vi "Teleop.vi"(10 "Match Info":T1={"Autonomous Elapsed Seconds"=0.0, "TeleOp Elapsed Seconds"=0.0, "Disabled Elapsed Seconds"=0.0, "Visited Autonomous"=FALSE, "Visited TeleOp"=FALSE, "Visited Disabled"=FALSE, "Autonomous Settings"={"Autonomous Style"=enum."Independent", "VI Refnum"=refnum}}, 11 "Call Context":T2) -> ()   [LabVIEW 2014]
doc: "This VI is called for each TeleOp packet received from the DS where the robot is not disabled. It is often used to read from the joysticks and update I/O or to update setpoints for timed control loops. It should complete and return within 20 milliseconds or it may miss DS packets."
uses:
  <vilib>/Rock Robotics/WPI/DriverStation/WPI_DriverStationDerivedRobotMode.ctl
  <vilib>/Rock Robotics/WPI/DriverStation/WPI_DriverStationMatch Info.ctl
  <vilib>/Rock Robotics/WPI/Joystick/WPI_JoystickGetSetRefNum.vi
  <vilib>/Rock Robotics/Network Tables/SD Write Boolean Array.vi
  <vilib>/Rock Robotics/Network Tables/SD Write Numeric Array.vi
  <vilib>/Rock Robotics/Network Tables/SD Read Boolean.vi
  <vilib>/Rock Robotics/Network Tables/SD Read Number.vi
  <vilib>/Rock Robotics/WPI/Solenoid/Deprecated/WPI_SolenoidSetBool.vi
  LIDAR Present Variable.vi
  <vilib>/functionblocks/Counter/Pulse Timer/Pulse Timer.vi
  <vilib>/Rock Robotics/WPI/RobotDrive/WPI_RobotDriveGetSetRefNum.vi
  <vilib>/Rock Robotics/WPI/RobotDrive/WPI_RobotDriveArcadeDrive_Standard(NoSaturation).vi
  <vilib>/functionblocks/Counter/Timer On Delay/Timer On Delay.vi
  <vilib>/functionblocks/FB Core/FB Core.xnode
  <vilib>/functionblocks/NI_FunctionBlock Libraries.lvlib
panel:
  out "Right Enc Status":string
  out "Right Enc Direction":string
  out "Right Encoder Rate":dbl
  out "Right Encoder Distance":dbl
  out "Left Enc Status":string
  out "Left Enc Direction":string
  out "Left Encoder Rate":dbl
  out "Left Encoder Distance":dbl
  out "Boolean 10":bool
  out "Boolean 9":bool
  out "Boolean 8":bool
  out "Boolean 7":bool
  out "Boolean 6":bool
  out "Boolean 5":bool
  out "Boolean 4":bool
  out "Boolean 3":bool
  out "Boolean 2":bool
  out "Boolean":bool
  out "Numeric 6":dbl
  out "Numeric 5":dbl
  out "Numeric 4":dbl
  out "Numeric 3":dbl
  out "Numeric 2":dbl
  out "Numeric":dbl
  out "Upper Roller Speed":dbl
  out "Arms Closed":bool
  out "Lidar (Inches)":dbl
  out "Arms Release":bool
  out "Lower PID Limit":dbl
  out "Upper PID Limit":dbl
  out "Upper Limit":bool
  out "Lower Limit":bool
  out "PID Input":dbl
  in  "Ext Dn Elv":bool
  in  "Ext Up Elv":bool
  out "Elevator Encoder":dbl(graph)
  out "Elevator Height":dbl
  out "Sample Slider 0":dbl(slide) scale=0.0..5.0
  out "Sample Boolean 1":bool
  out "Sample Boolean 0":bool
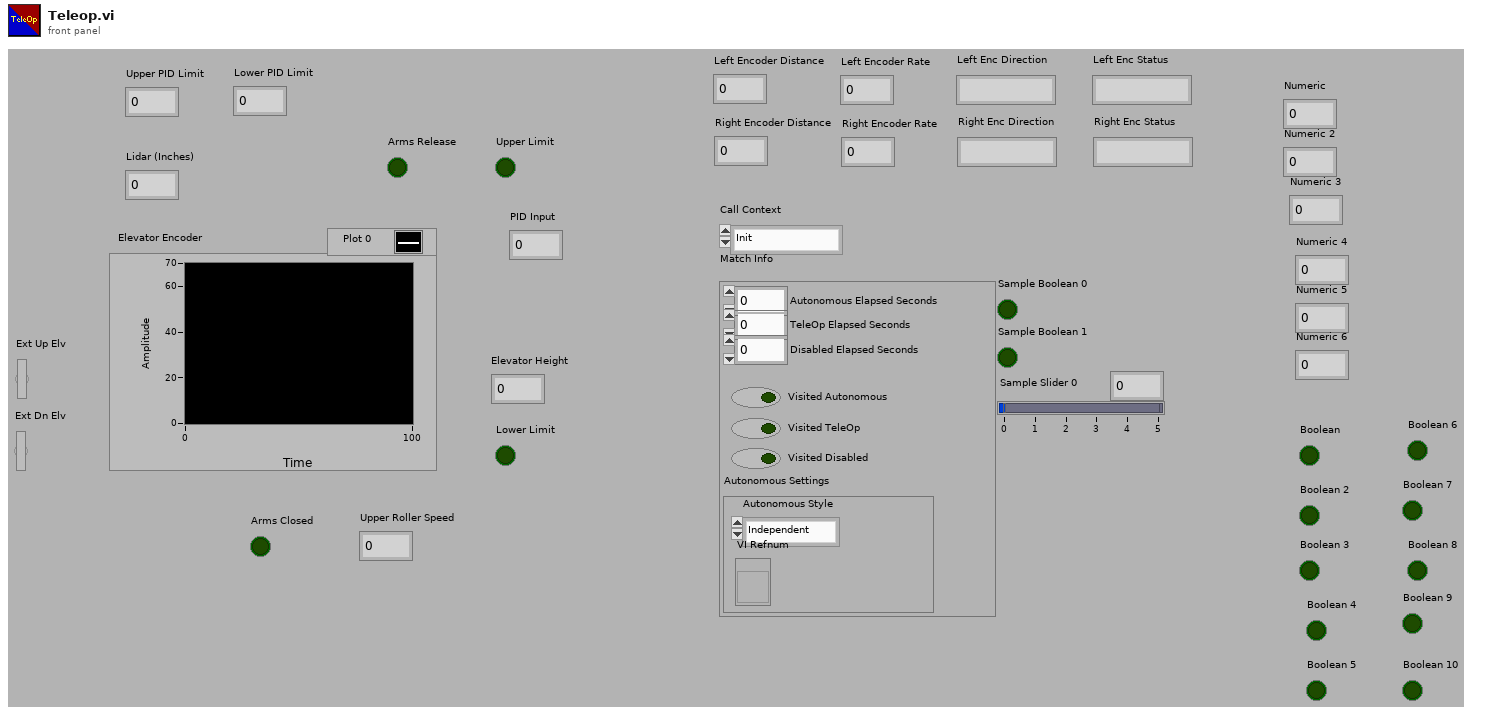
[diagram p1: front panel]
types:
  T1 = typedef "WPI_DriverStationMatch Info.ctl" = cluster{"Autonomous Elapsed Seconds":dbl, "TeleOp Elapsed Seconds":dbl, "Disabled Elapsed Seconds":dbl, "Visited Autonomous":bool, "Visited TeleOp":bool, "Visited Disabled":bool, "Autonomous Settings":cluster{"Autonomous Style":enum16{"Iterative", "Independent"}, "VI Refnum":refnum<vi>}}
  T2 = typedef "WPI_DriverStationDerivedRobotMode.ctl" = enum16{"Init", "Execute", "Stop"}
  T3 = typedef "WPI_JoystickDevRef.ctl" = cluster{"Device":T4}
  T4 = typedef "WPI_JoystickDeviceEnum.ctl" = enum16{"USB 0", "USB 1", "USB 2", "USB 3", "USB 4", "USB 5"}
  T5 = typedef "WPI_I2CDevRef.ctl" = cluster{"DevStatus":errorcluster, "Controller":T6, "Device Address":u8, "Handle":i32, "I2C Bus":T7}
  T6 = typedef "FPGA_TypedefDigitalModule.ctl" = enum16{"Controller 1"}
  T7 = typedef "i2c_bus.ctl" = enum16{"I2C On-Board", "I2C MXP", "Invalid"}
  T8 = cluster{bool, bool, "Ext Up Elv":bool, "Ext Dn Elv":bool, bool, bool}
  T9 = typedef "WPI_EncoderDevRef.ctl" = cluster{"DevStatus":errorcluster, "EncoderIndex":T10, "CounterIndex":T11, "DistancePerCount":dbl, "Decoding Type":T12}
  T10 = typedef "FPGA_EncoderIdx.ctl" = enum8{"Enc 0", "Enc 1", "Enc 2", "Enc 3", "Enc 4", "Enc 5", "Enc 6", "Enc 7", "Invalid"}
  T11 = typedef "FPGA_CounterCtrSystemIndex.ctl" = enum8{"Ctr 0", "Ctr 1", "Ctr 2", "Ctr 3", "Ctr 4", "Ctr 5", "Ctr 6", "Ctr 7", "Invalid"}
  T12 = typedef "WPI_EncoderType.ctl" = enum16{"1x", "2x", "4x"}
  T13 = typedef "WPI_SolenoidDevRef.ctl" = cluster{"DevStatus":errorcluster, "Pneumatics Control Module":u8, "Forward Solenoid Channel":T14, "Reverse Solenoid Channel":T14}
  T14 = typedef "WPI_SolenoidChannel.ctl" = enum8{"Solenoid 0", "Solenoid 1", "Solenoid 2", "Solenoid 3", "Solenoid 4", "Solenoid 5", "Solenoid 6", "Solenoid 7", "Invalid"}
  T15 = typedef "WPI_RobotDriveDevRef.ctl" = cluster{"DevStatus":errorcluster, "Motors[]":T16[], "Square Inputs":bool, "Max Output":dbl}
  T16 = typedef "WPI_MotorControlDeviceRef.ctl" = cluster{"DeviceStatus":errorcluster, "Type":T17, "PWM":cluster{"Controller":T6, "PWM Channel":T18, "DeadBand":T19}, "CAN":cluster{"Device Number":u8, "Control Mode":T20, "Semaphore":T21, "Max Vout":dbl, "TalonSRX Control Mode":T22}, "Invert":bool, "TransformRef":T23, "InvTransformRef":T23}
  T17 = typedef "WPI_MotorControlType.ctl" = enum16{"PWM", "CAN", "CANTalonSRX"}
  T18 = typedef "FPGA_DIOPWMChannel.ctl" = enum8{"PWM 0", "PWM 1", "PWM 2", "PWM 3", "PWM 4", "PWM 5", "PWM 6", "PWM 7", "PWM 8", "PWM 9", "PWM MXP 0", "PWM MXP 1", "PWM MXP 2", "PWM MXP 3", "PWM MXP 4", "PWM MXP 5", "PWM MXP 6", "PWM MXP 7", "PWM MXP 8", "PWM MXP 9", "Invalid"}
  T19 = typedef "WPI_PWMDeadband.ctl" = cluster{"Name":string, "maxPositivePwm":i32, "minPositivePwm":i32, "centerPwm":i32, "maxNegativePwm":i32, "minNegativePwm":i32, "angularRange":u16}
  T20 = typedef "WPI_CANJaguar_ControlMode.ctl" = enum8{"Percent VBus", "Current", "Speed", "Position", "Voltage"}
  T21 = typedef "Semaphore RefNum" = refnum<k1>
  T22 = typedef "WPI_CANTalonSRX_APIControlMode.ctl" = enum8{"Percent VBus", "Speed", "Position", "Slave", "Unchanged / Invalid"}
  T23 = typedef "WPI_PWMTransform_ConPane.ctl" = refnum<vi>
  T24 = typedef "WPI_DigitalInputDevRef.ctl" = cluster{"DevStatus":errorcluster, "DIO Channel":T25, "Controller":T6}
  T25 = typedef "FPGA_DIOChannel.ctl" = enum8{"DIO 0", "DIO 1", "DIO 2", "DIO 3", "DIO 4", "DIO 5", "DIO 6", "DIO 7", "DIO 8", "DIO 9", "DIO MXP 0", "DIO MXP 1", "DIO MXP 2", "DIO MXP 3", "DIO MXP 4", "DIO MXP 5", "DIO MXP 6", "DIO MXP 7", "DIO MXP 8", "DIO MXP 9", "DIO MXP 10", "DIO MXP 11", "DIO MXP 12", "DIO MXP 13", "DIO MXP 14", "DIO MXP 15", "Invalid"}
  T26 = cluster{"Upper Value ":dbl, "Upper Max Speed ":dbl, "Encoder Distance":dbl, "Slowdown":dbl, "Lower Value":dbl, "Value":bool, "Value":bool, "Lower Max Speed":dbl}
  T27 = cluster{"Elevator Final Reference":dbl, "Enc Offset":dbl, "Value":bool}
  T28 = cluster{"Encoder Alarm Status":string, "Encoder Distance":dbl, "Encoder Direction":string, "Encoder Rate (distance/sec)":dbl}
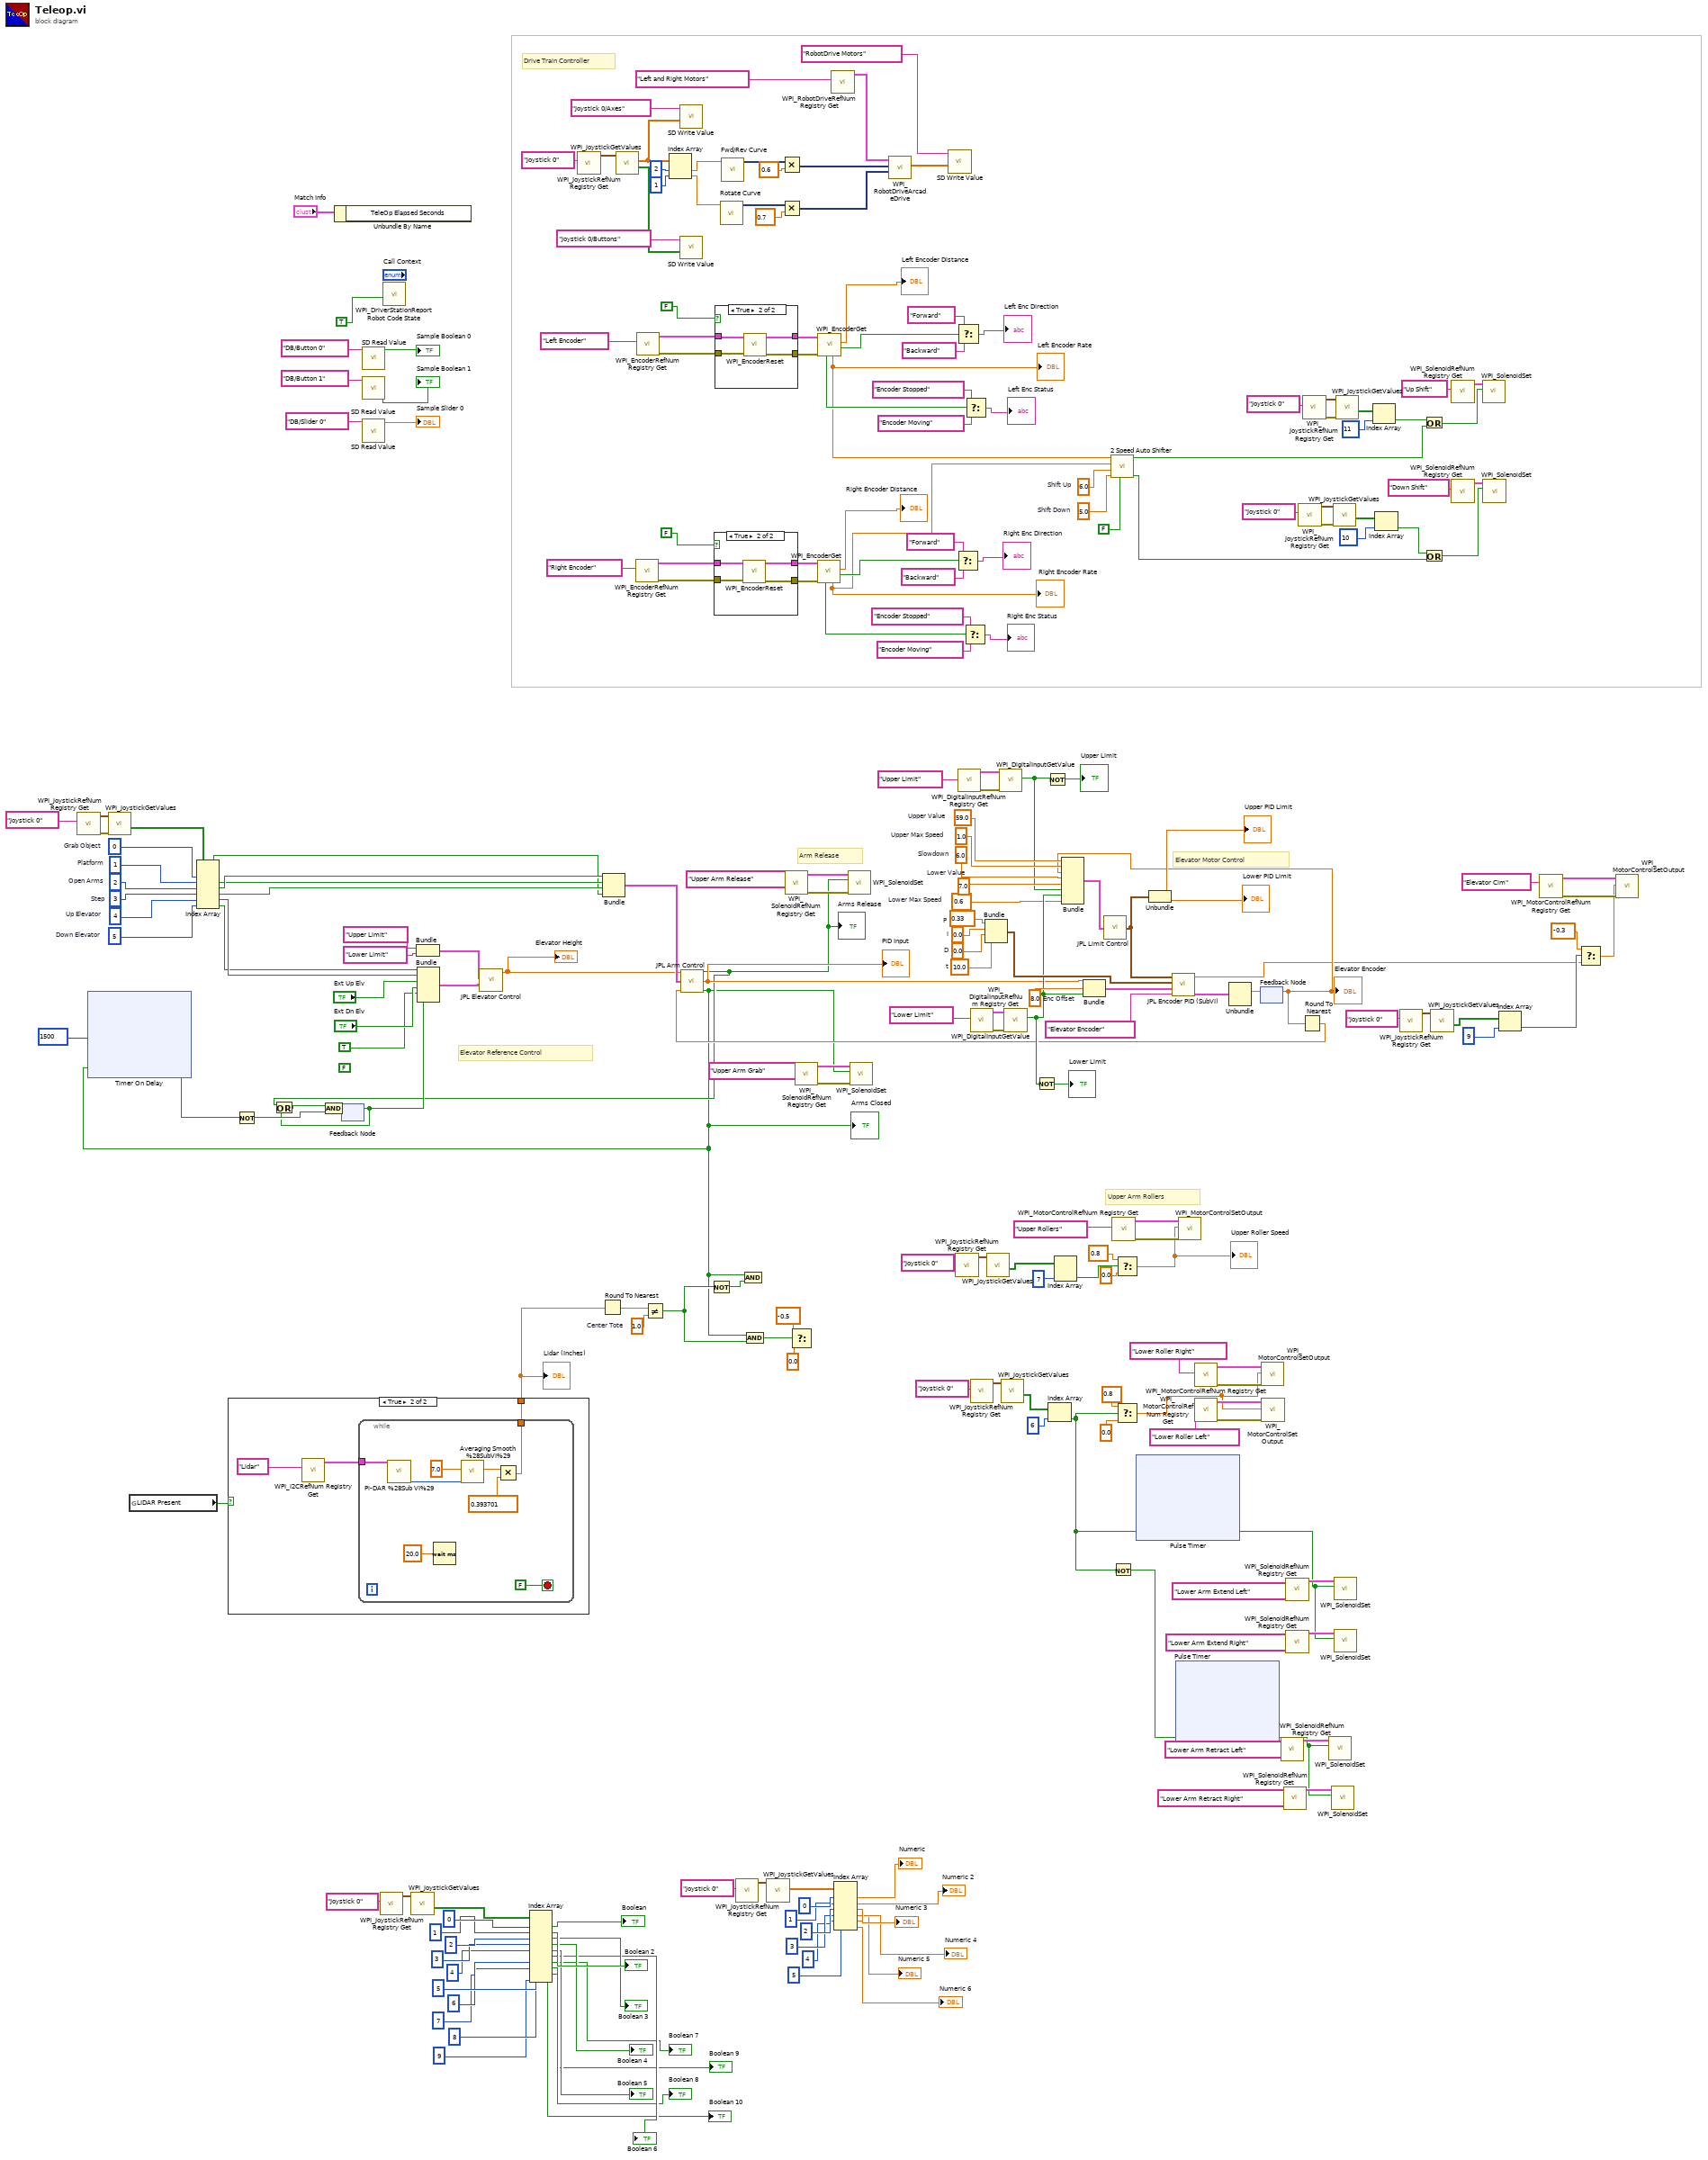
[diagram p0: block diagram]
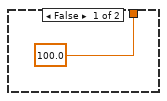
[diagram p4: hidden frame]
diagram:
  w2 = 5.0  # Shift Down
  w3 = 6.0  # Shift Up
  (unwired) FALSE
  w144 = 0.6  # Lower Max Speed
  w172 = 1.0  # Center Tote
  w175 = 7.0  # Lower Value
  w178 = 59.0  # Upper Value
  w196 = 5  # Down Elevator
  w197 = 4  # Up Elevator
  w198 = 3  # Step
  w199 = 2  # Open Arms
  w187 = 8.0  # Enc Offset
  w189 = 10.0  # t
  w203 = 0.0  # D
  w204 = 0.0  # I
  w205 = 0.33  # P
  w176 = 6.0  # Slowdown
  w177 = 1.0  # Upper Max Speed
  w206 = 1  # Platform
  w208 = 0  # Grab Object
  # "Upper Arm Rollers"
  # "Arm Release"
  # "Elevator Reference Control"
  # "Elevator Motor Control"
  # "Drive Train Controller"
  n1 = call <vilib>:"WPI_JoystickRefNum Registry Get.vi"("refnum name"="Joystick 0") -> ("error out"=w209:errorcluster, "JoystickDevRef"=w210:T3)  [unwired: 1 in, 8 out]
  n2 = call <vilib>:"WPI_JoystickGetValues.vi"("error in (no error)"=w209, "JoystickDevRef"=w210) -> ("Buttons"=w207:bool[])  [unwired: 5 in, 4 out]
  n3 = global read "LIDAR Present Variable.vi" "LIDAR Present"() -> (w184:bool)
  n4 = Index Array(array=w207, index #1=w208, index #2=w206, index #3=w199, index #4=w198, index #5=w197, index #6=w196) -> (element #1=w50:bool, element #2=w52:bool, element #3=w53:bool, element #4=w51:bool, element #5=w152:bool, element #6=w151:bool)
  n5 = case shown="True" w184 {
    tunnel: [100.0 w250] -> w154
    frame False {
    }
    frame True {
      n6 = call <vilib>:"WPI_I2CRefNum Registry Get.vi"("refnum name"="Lidar") -> ("I2CDevRef"=w251:T5)  [unwired: 9 in, 1 out]
      n7 = while {
        tunnel: w251 -> [w256]
        tunnel: [w253] -> w250
        stop <- FALSE stop-if-true
        n8 = call "Pi-DAR %28Sub VI%29.vi"("I2CDevRef"=w256) -> ("Distance Output"=w260:i32)  [unwired: 10 in]
        n9 = Wait (ms)(milliseconds to wait=20.0) -> ()  [unwired: 1 out]
        n10 = call "Averaging Smooth %28SubVI%29.vi"("Input"=w260, "# of Samples to Average"=7.0) -> ("Output"=w255:dbl)  [unwired: 6 in, 1 out]
        n11 = Multiply(x=w255, y=0.393701) -> (x*y=w253:dbl)
      }
    }
  }
  "Lidar (Inches)" <- w154
  n12 = Unbundle By Name("Match Info") -> ()  [unwired: 1 out]
  n13 = feedback #1() -> (w16:bool)  [unwired: 1 in]
  n14 = call-poly <vilib>:"SD Read Value.vi"("Name"="DB/Button 0" ("refnum name")) -> ("Boolean"=→"Sample Boolean 0":bool)  [unwired: 8 in, 2 out]
  n15 = call-poly <vilib>:"SD Read Value.vi"("Name"="DB/Button 1" ("refnum name")) -> ("Boolean"=→"Sample Boolean 1":bool)  [unwired: 8 in, 2 out]
  n16 = call-poly <vilib>:"SD Read Value.vi"("Name"="DB/Slider 0" ("refnum name")) -> ("Numeric"=→"Sample Slider 0":dbl)  [unwired: 8 in, 2 out]
  n17 = call <vilib>:"WPI_JoystickRefNum Registry Get.vi"("refnum name"="Joystick 0") -> ("JoystickDevRef"=w127:T3)  [unwired: 1 in, 9 out]
  n18 = call <vilib>:"WPI_DriverStationReport Robot Code State.vi"("TeleOp"=TRUE ("Autonomous")) -> ()  [unwired: 10 in, 1 out]
  n19 = call <vilib>:"WPI_JoystickGetValues.vi"("JoystickDevRef"=w127) -> ("Buttons"=w120:bool[])  [unwired: 6 in, 4 out]
  n20 = Bundle("Upper Limit", "Lower Limit") -> (w195:cluster{string, string})  [unwired: 1 in]
  n21 = Bundle(w151, w152, "Ext Up Elv"="Ext Up Elv", "Ext Dn Elv"="Ext Dn Elv", TRUE, w16) -> (w192:T8)  [unwired: 1 in]
  n22 = call "JPL Elevator Control.vi"("Button Control"=w192, "Limit Switches"=w195) -> ("Elevator Height"=w47:dbl)  [unwired: 8 in, 1 out]
  "Elevator Height" <- w47
  n23 = Index Array(array=w120, index #1=0, index #2=1, index #3=2, index #4=3, index #5=4, index #6=5, index #7=6, index #8=7, index #9=8, index #10=9) -> (element #1=→"Boolean":bool, element #2=→"Boolean 2":bool, element #3=→"Boolean 3":bool, element #4=→"Boolean 4":bool, element #5=→"Boolean 5":bool, element #6=→"Boolean 6":bool, element #7=→"Boolean 7":bool, element #8=→"Boolean 8":bool, element #9=→"Boolean 9":bool, element #10=→"Boolean 10":bool)
  n24 = call <vilib>:"WPI_JoystickRefNum Registry Get.vi"("refnum name"="Joystick 0") -> ("JoystickDevRef"=w244:T3)  [unwired: 1 in, 9 out]
  n25 = Round To Nearest(number=w154) -> (nearest integer value=w155:dbl)
  n26 = Bundle(w53, w52, w51, w50) -> (w54:cluster{bool, bool, bool, bool})  [unwired: 1 in]
  n27 = call <vilib>:"WPI_JoystickGetValues.vi"("JoystickDevRef"=w244) -> ("Buttons"=w234:bool[], "Axes"=w236:dbl[])  [unwired: 6 in, 3 out]
  n28 = call <vilib>:"WPI_EncoderRefNum Registry Get.vi"("refnum name"="Right Encoder" ("Name")) -> ("error out"=w72:errorcluster, "EncoderDevRef"=w71:T9)  [unwired: 9 in]
  n29 = call <vilib>:"WPI_EncoderRefNum Registry Get.vi"("refnum name"="Left Encoder" ("Name")) -> ("error out"=w87:errorcluster, "EncoderDevRef"=w86:T9)  [unwired: 9 in]
  n30 = Not Equal?(x=w155, y=w172) -> (x != y?=w164:bool)
  n31 = Index Array(array=w236, index #1=2, index #2=1) -> (element #1=w57:dbl, element #2=w97:dbl)
  n32 = call-poly <vilib>:"SD Write Value.vi"("Numeric Array"=w236, "Name"="Joystick 0/Axes") -> ()  [unwired: 8 in, 2 out]
  n33 = call-poly <vilib>:"SD Write Value.vi"("Boolean Array"=w234, "Name"="Joystick 0/Buttons") -> ()  [unwired: 8 in, 2 out]
  n34 = Not(x=w164) -> (.not. x?=w163:bool)
  n35 = case shown="True" FALSE {
    tunnel: w71 -> [w262 w263]
    tunnel: [w262 w266] -> w73
    tunnel: w72 -> [w261 w265]
    tunnel: [w261 w264] -> w80
    frame False {
    }
    frame True {
      n36 = call <vilib>:"WPI_EncoderReset.vi"("error in (no error)"=w265, "EncoderDevRef"=w263) -> ("error out"=w264:errorcluster, "EncoderDevRef"=w266:T9)  [unwired: 8 out]
    }
  }
  n37 = case shown="True" FALSE {
    tunnel: w86 -> [w268 w269]
    tunnel: [w268 w272] -> w88
    tunnel: w87 -> [w267 w271]
    tunnel: [w267 w270] -> w95
    frame False {
    }
    frame True {
      n38 = call <vilib>:"WPI_EncoderReset.vi"("error in (no error)"=w271, "EncoderDevRef"=w269) -> ("error out"=w270:errorcluster, "EncoderDevRef"=w272:T9)  [unwired: 8 out]
    }
  }
  n39 = call "Rotate Curve"("Signals"=w97) -> ("Scaled Signals"=w96:dynamicdata)  [unwired: 9 in, 1 out]
  n40 = call "Fwd/Rev Curve"("Signals"=w57) -> ("Scaled Signals"=w98:dynamicdata)  [unwired: 9 in, 1 out]
  n41 = call <vilib>:"WPI_JoystickRefNum Registry Get.vi"("refnum name"="Joystick 0") -> ("JoystickDevRef"=w142:T3)  [unwired: 1 in, 9 out]
  n42 = call <vilib>:"WPI_JoystickGetValues.vi"("JoystickDevRef"=w142) -> ("Axes"=w141:dbl[])  [unwired: 6 in, 4 out]
  n43 = Multiply(x=w98, y=0.6) -> (x*y=w55:dynamicdata)
  n44 = Multiply(x=w96, y=0.7) -> (x*y=w56:dynamicdata)
  n45 = call <vilib>:"WPI_SolenoidRefNum Registry Get.vi"("refnum name"="Upper Arm Release") -> ("error out"=w160:errorcluster, "SolenoidDevRef"=w162:T13)  [unwired: 9 in]
  n46 = call <vilib>:"WPI_SolenoidRefNum Registry Get.vi"("refnum name"="Upper Arm Grab") -> ("error out"=w170:errorcluster, "SolenoidDevRef"=w174:T13)  [unwired: 9 in]
  n47 = call <vilib>:"WPI_EncoderGet.vi"("error in (no error)"=w80, "EncoderDevRef"=w73) -> ("Direction"=w74:bool, "Distance"=→"Right Encoder Distance":dbl, "Rate"=w6:dbl, "Stopped"=w75:bool)  [unwired: 6 out]
  "Right Encoder Rate" <- w6
  n48 = call <vilib>:"WPI_EncoderGet.vi"("error in (no error)"=w95, "EncoderDevRef"=w88) -> ("Direction"=w89:bool, "Distance"=→"Left Encoder Distance":dbl, "Rate"=w7:dbl, "Stopped"=w90:bool)  [unwired: 6 out]
  "Left Encoder Rate" <- w7
  n49 = call <vilib>:"WPI_RobotDriveRefNum Registry Get.vi"("refnum name"="Left and Right Motors") -> ("RobotDriveDevRef"=w246:T15)  [unwired: 1 in, 9 out]
  n50 = Index Array(array=w141, index #1=0, index #2=1, index #3=2, index #4=3, index #5=4, index #6=5) -> (element #1=→"Numeric":dbl, element #2=→"Numeric 2":dbl, element #3=→"Numeric 3":dbl, element #4=→"Numeric 4":dbl, element #5=→"Numeric 5":dbl, element #6=→"Numeric 6":dbl)
  n51 = call-poly <vilib>:"WPI_RobotDriveArcadeDrive.vi"("Y axis value"=w56, "X axis value"=w55, "RobotDriveDevRef"=w246) -> ("Motor Values"=w238:dbl[])  [unwired: 6 in, 2 out]
  n52 = call-poly <vilib>:"SD Write Value.vi"("Numeric Array"=w238, "Name"="RobotDrive Motors") -> ()  [unwired: 8 in, 2 out]
  n53 = call <vilib>:"WPI_JoystickRefNum Registry Get.vi"("refnum name"="Joystick 0") -> ("JoystickDevRef"=w149:T3)  [unwired: 1 in, 9 out]
  n54 = Select(t="Forward", s=w74, f="Backward") -> (s? t:f=→"Right Enc Direction":string)
  n55 = Select(t="Forward", s=w89, f="Backward") -> (s? t:f=→"Left Enc Direction":string)
  n56 = call <vilib>:"WPI_DigitalInputRefNum Registry Get.vi"("refnum name"="Upper Limit") -> ("error out"=w182:errorcluster, "DigitalInputDevRef"=w183:T24)  [unwired: 9 in]
  n57 = Select(t="Encoder Stopped", s=w75, f="Encoder Moving") -> (s? t:f=→"Right Enc Status":string)
  n58 = Select(t="Encoder Stopped", s=w90, f="Encoder Moving") -> (s? t:f=→"Left Enc Status":string)
  n59 = call <vilib>:"WPI_DigitalInputRefNum Registry Get.vi"("refnum name"="Lower Limit") -> ("error out"=w212:errorcluster, "DigitalInputDevRef"=w214:T24)  [unwired: 9 in]
  n60 = call <vilib>:"WPI_JoystickRefNum Registry Get.vi"("refnum name"="Joystick 0") -> ("JoystickDevRef"=w44:T3)  [unwired: 1 in, 9 out]
  n61 = Bundle("P"=w205, "I"=w204, "D"=w203, "t"=w189) -> (w190:cluster{"P":dbl, "I":dbl, "D":dbl, "t":dbl})  [unwired: 1 in]
  n62 = call <vilib>:"WPI_JoystickGetValues.vi"("JoystickDevRef"=w149) -> ("Buttons"=w104:bool[])  [unwired: 6 in, 4 out]
  n63 = call <vilib>:"WPI_DigitalInputGetValue.vi"("error in (no error)"=w182, "DigitalInputDevRef"=w183) -> ("Value"=w147:bool)  [unwired: 7 in, 2 out]
  n64 = call <vilib>:"WPI_JoystickGetValues.vi"("JoystickDevRef"=w44) -> ("Buttons"=w43:bool[])  [unwired: 6 in, 4 out]
  n65 = call <vilib>:"WPI_DigitalInputGetValue.vi"("error in (no error)"=w212, "DigitalInputDevRef"=w214) -> ("Value"=w145:bool)  [unwired: 7 in, 2 out]
  n66 = Not(x=w145) -> (.not. x?=→"Lower Limit":bool)
  n67 = Not(x=w147) -> (.not. x?=→"Upper Limit":bool)
  n68 = Index Array(array=w43, index=6) -> (element=w22:bool)
  n69 = Index Array(array=w104, index #2=7) -> (element #2=w101:bool)  [unwired: 1 in, 1 out]
  n70 = call "2 Speed Auto Shifter.vi"("Enable"=FALSE, "Down Shift Value"=w2, "Up Shift Value"=w3, "Right Enc Rate"=w6, "Left  Enc Rate"=w7) -> ("Down Shift"=w5:bool, "Up Shift"=w4:bool)  [unwired: 4 in]
  n71 = Not(x=w22) -> (.not. x?=w21:bool)
  n72 = call <vilib>:"WPI_MotorControlRefNum Registry Get.vi"("refnum name"="Upper Rollers") -> ("error out"=w167:errorcluster, "MotorControlDevRef"=w168:T16)  [unwired: 9 in]
  n73 = Select(t=0.8, s=w101, f=0.0) -> (s? t:f=w33:dbl)
  "Upper Roller Speed" <- w33
  n74 = Select(t=0.8, s=w22, f=0.0) -> (s? t:f=w32:dbl)
  n75 = xnode "Pulse Timer"("input"=w22) -> ("output"=w23:bool)  [unwired: 2 in, 2 out]
  n76 = xnode "Pulse Timer"("input"=w21) -> ("output"=w20:bool)  [unwired: 2 in, 2 out]
  n77 = call <vilib>:"WPI_MotorControlSetOutput.vi"("error in (no error)"=w167, "Output"=w33, "MotorControlDevRef"=w168) -> ()  [unwired: 6 in, 3 out]
  n78 = call <vilib>:"WPI_MotorControlRefNum Registry Get.vi"("refnum name"="Lower Roller Right") -> ("error out"=w36:errorcluster, "MotorControlDevRef"=w37:T16)  [unwired: 9 in]
  n79 = call <vilib>:"WPI_MotorControlRefNum Registry Get.vi"("refnum name"="Lower Roller Left") -> ("error out"=w38:errorcluster, "MotorControlDevRef"=w39:T16)  [unwired: 9 in]
  n80 = feedback #2() -> (w153:dbl)  [unwired: 1 in]
  "Elevator Encoder" <- w153
  n81 = Bundle("Upper Value"=w178, "Upper Max Speed"=w177, "Encoder Distance"=w153, "Slowdown"=w176, "Lower Value"=w175, "Value"=w147, "Value"=w145, "Lower Max Speed"=w144) -> (w157:T26)  [unwired: 1 in]
  n82 = call "JPL Limit Control.vi"("Limit Inputs"=w157) -> ("Limit Output"=w156:cluster{"Positive Out":dbl, "Negative Out":dbl})  [unwired: 4 in]
  n83 = Unbundle(w156) -> ("Positive Out"=→"Upper PID Limit":dbl, "Negative Out"=→"Lower PID Limit":dbl)
  n84 = call <vilib>:"WPI_MotorControlSetOutput.vi"("error in (no error)"=w36, "Output"=w32, "MotorControlDevRef"=w37) -> ()  [unwired: 6 in, 3 out]
  n85 = call <vilib>:"WPI_MotorControlSetOutput.vi"("error in (no error)"=w38, "Output"=w32, "MotorControlDevRef"=w39) -> ()  [unwired: 6 in, 3 out]
  n86 = call <vilib>:"WPI_SolenoidRefNum Registry Get.vi"("refnum name"="Lower Arm Retract Left") -> ("SolenoidDevRef"=w30:T13)  [unwired: 9 in, 1 out]
  n87 = call <vilib>:"WPI_SolenoidRefNum Registry Get.vi"("refnum name"="Lower Arm Retract Right") -> ("SolenoidDevRef"=w26:T13)  [unwired: 9 in, 1 out]
  n88 = call <vilib>:"WPI_SolenoidRefNum Registry Get.vi"("refnum name"="Lower Arm Extend Left") -> ("SolenoidDevRef"=w31:T13)  [unwired: 9 in, 1 out]
  n89 = call <vilib>:"WPI_SolenoidRefNum Registry Get.vi"("refnum name"="Lower Arm Extend Right") -> ("SolenoidDevRef"=w27:T13)  [unwired: 9 in, 1 out]
  n90 = call <vilib>:"WPI_JoystickRefNum Registry Get.vi"("refnum name"="Joystick 0") -> ("error out"=w220:errorcluster, "JoystickDevRef"=w221:T3)  [unwired: 1 in, 8 out]
  n91 = Round To Nearest(number=w153) -> (nearest integer value=w49:dbl)
  n92 = call "JPL Arm Control.vi"("Elevator Array"=w47, "Joystick Boolean Inputs"=w54, "Actual Height"=w49) -> ("Arms Release"=w15:bool, "Elevator Final Reference"=w48:dbl, "Arms Closed"=w14:bool)  [unwired: 10 in]
  "PID Input" <- w48
  "Arms Release" <- w15
  "Arms Closed" <- w14
  n93 = xnode "Timer On Delay"("preset time (ms)"=1500, "input"=w14) -> ("output"=w13:bool)  [unwired: 1 in, 2 out]
  n94 = Not(x=w13) -> (.not. x?=w17:bool)
  n95 = Or(x=w15, y=w16) -> (x .or. y?=w19:bool)
  n96 = And(x=w19, y=w17) -> (x .and. y?=w18:bool)
  n97 = feedback-in #1(w18) -> ()
  n98 = And(x=w14, y=w163) -> ()  [unwired: 1 out]
  n99 = And(x=w14, y=w164) -> (x .and. y?=w171:bool)
  n100 = Select(t=-0.5, s=w171, f=0.0) -> ()  [unwired: 1 out]
  n101 = call-poly <vilib>:"WPI_SolenoidSet.vi"("error in (no error)"=w160, "Value"=w15, "SolenoidDevRef"=w162) -> ()  [unwired: 7 in, 2 out]
  n102 = call-poly <vilib>:"WPI_SolenoidSet.vi"("error in (no error)"=w170, "Value"=w14, "SolenoidDevRef"=w174) -> ()  [unwired: 7 in, 2 out]
  n103 = Bundle("Elevator Final Reference"=w48, "Enc Offset"=w187, "Value"=w145) -> (w188:T27)  [unwired: 1 in]
  n104 = call "JPL Encoder PID (SubVI).vi"("refnum name"="Elevator Encoder", "Encoder Config"=w188, "PID Settings"=w190, "PID Limits"=w156) -> ("Encoder Status"=w186:T28, "output"=w59:dbl)  [unwired: 2 in]
  n105 = Unbundle(w186) -> ("Encoder Distance"=w185:dbl)  [unwired: 3 out]
  n106 = feedback-in #2(w185) -> ()
  n107 = call <vilib>:"WPI_JoystickRefNum Registry Get.vi"("refnum name"="Joystick 0") -> ("error out"=w226:errorcluster, "JoystickDevRef"=w227:T3)  [unwired: 1 in, 8 out]
  n108 = call-poly <vilib>:"WPI_SolenoidSet.vi"("Value"=w20, "SolenoidDevRef"=w30) -> ()  [unwired: 8 in, 2 out]
  n109 = call-poly <vilib>:"WPI_SolenoidSet.vi"("Value"=w20, "SolenoidDevRef"=w26) -> ()  [unwired: 8 in, 2 out]
  n110 = call <vilib>:"WPI_JoystickGetValues.vi"("error in (no error)"=w220, "JoystickDevRef"=w221) -> ("Buttons"=w219:bool[])  [unwired: 5 in, 4 out]
  n111 = call-poly <vilib>:"WPI_SolenoidSet.vi"("Value"=w23, "SolenoidDevRef"=w31) -> ()  [unwired: 8 in, 2 out]
  n112 = call-poly <vilib>:"WPI_SolenoidSet.vi"("Value"=w23, "SolenoidDevRef"=w27) -> ()  [unwired: 8 in, 2 out]
  n113 = call <vilib>:"WPI_JoystickGetValues.vi"("error in (no error)"=w226, "JoystickDevRef"=w227) -> ("Buttons"=w225:bool[])  [unwired: 5 in, 4 out]
  n114 = Index Array(array=w225, index=11) -> (element=w11:bool)
  n115 = Index Array(array=w219, index=10) -> (element=w8:bool)
  n116 = call <vilib>:"WPI_JoystickRefNum Registry Get.vi"("refnum name"="Joystick 0") -> ("JoystickDevRef"=w64:T3)  [unwired: 1 in, 9 out]
  n117 = Or(x=w11, y=w4) -> (x .or. y?=w10:bool)
  n118 = Or(x=w8, y=w5) -> (x .or. y?=w9:bool)
  n119 = call <vilib>:"WPI_JoystickGetValues.vi"("JoystickDevRef"=w64) -> ("Buttons"=w62:bool[])  [unwired: 6 in, 4 out]
  n120 = call <vilib>:"WPI_SolenoidRefNum Registry Get.vi"("refnum name"="Up Shift") -> ("SolenoidDevRef"=w224:T13)  [unwired: 9 in, 1 out]
  n121 = call <vilib>:"WPI_SolenoidRefNum Registry Get.vi"("refnum name"="Down Shift") -> ("SolenoidDevRef"=w218:T13)  [unwired: 9 in, 1 out]
  n122 = call-poly <vilib>:"WPI_SolenoidSet.vi"("Value"=w10, "SolenoidDevRef"=w224) -> ()  [unwired: 8 in, 2 out]
  n123 = call-poly <vilib>:"WPI_SolenoidSet.vi"("Value"=w9, "SolenoidDevRef"=w218) -> ()  [unwired: 8 in, 2 out]
  n124 = Index Array(array=w62, index=9) -> (element=w61:bool)
  n125 = call <vilib>:"WPI_MotorControlRefNum Registry Get.vi"("refnum name"="Elevator Cim") -> ("error out"=w201:errorcluster, "MotorControlDevRef"=w202:T16)  [unwired: 9 in]
  n126 = Select(t=-0.3, s=w61, f=w59) -> (s? t:f=w58:dbl)
  n127 = call <vilib>:"WPI_MotorControlSetOutput.vi"("error in (no error)"=w201, "Output"=w58, "MotorControlDevRef"=w202) -> ()  [unwired: 6 in, 3 out]
